vi "Up_PatternMatch.vi"(0 "Image In":T4, 2 "Template Image":T4, 5 "ROIIn":string, 11 "error in":errorcluster) -> (3 "Match":T1, 4 "Image Out":T4, 6 "Result":T3, 8 "ResultShow":T2, 10 "OK":bool, 14 "resulting string":string, 15 "error out":errorcluster)   [LabVIEW 2019]
uses:
  <vilib>/vision/Image Controls.llb/IMAQ Image.ctl
  <vilib>/vision/NI_Vision_Development_Module.lvlib
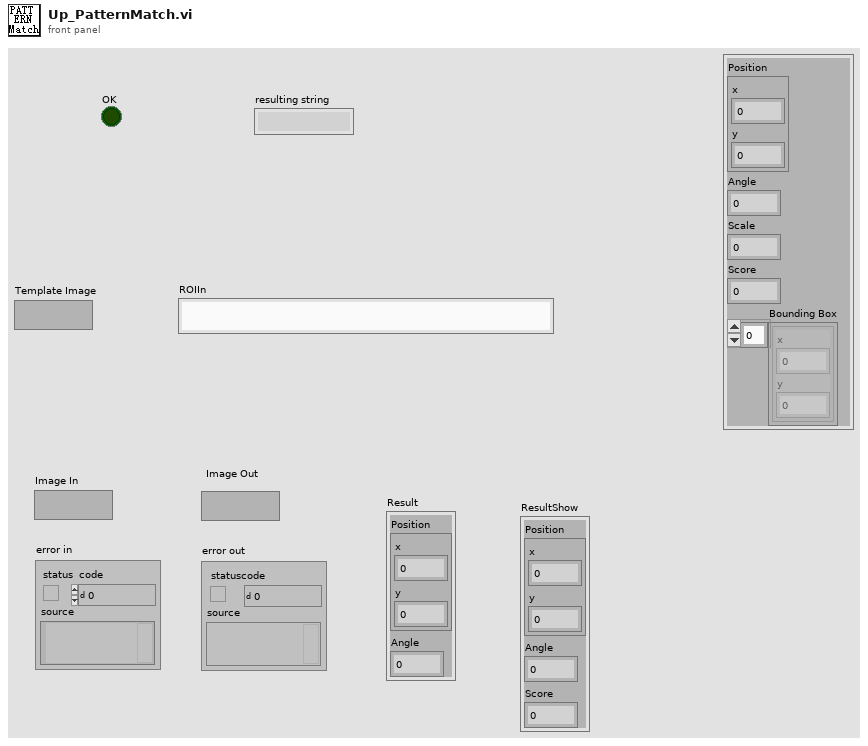
[diagram p1: front panel]
types:
  T1 = cluster{"Position":cluster{"x":sgl, "y":sgl}, "Angle":sgl, "Scale":sgl, "Score":sgl, "Bounding Box":cluster{"x":sgl, "y":sgl}[]}
  T2 = cluster{"Position":cluster{"x":sgl, "y":sgl}, "Angle":sgl, "Score":sgl}
  T3 = cluster{"Position":cluster{"x":sgl, "y":sgl}, "Angle":sgl}
  T4 = typedef "IMAQ Image.ctl" = refnum<image>
  T5 = typedef "IMAQ Rectangle" = cluster{"Left":i32, "Top":i32, "Right":i32, "Bottom":i32, "Rotation":dbl}
  T6 = cluster{"Number of Matches Requested":i32, "Minimum Match Score":sgl, "Angle Ranges":cluster{"Start Angle":sgl, "End Angle":sgl}[]}
  T7 = typedef "Image Type" = u32
  T8 = typedef "ROI Descriptor" = cluster{"Global Rectangle":i32[], "Contours":cluster{"ID":enum32{"External", "Internal"}, "Type":u32, "Coordinates":i32[]}[]}
  T9 = cluster{"Position":cluster{"x":sgl, "y":sgl}, "Angle":sgl, "Scale":sgl, "Score":sgl, "Bounding Box":cluster{"x":sgl, "y":sgl}[]}[]
  T10 = cluster{"Position":cluster{"x":sgl, "y":sgl}, "Angle":sgl, sgl}
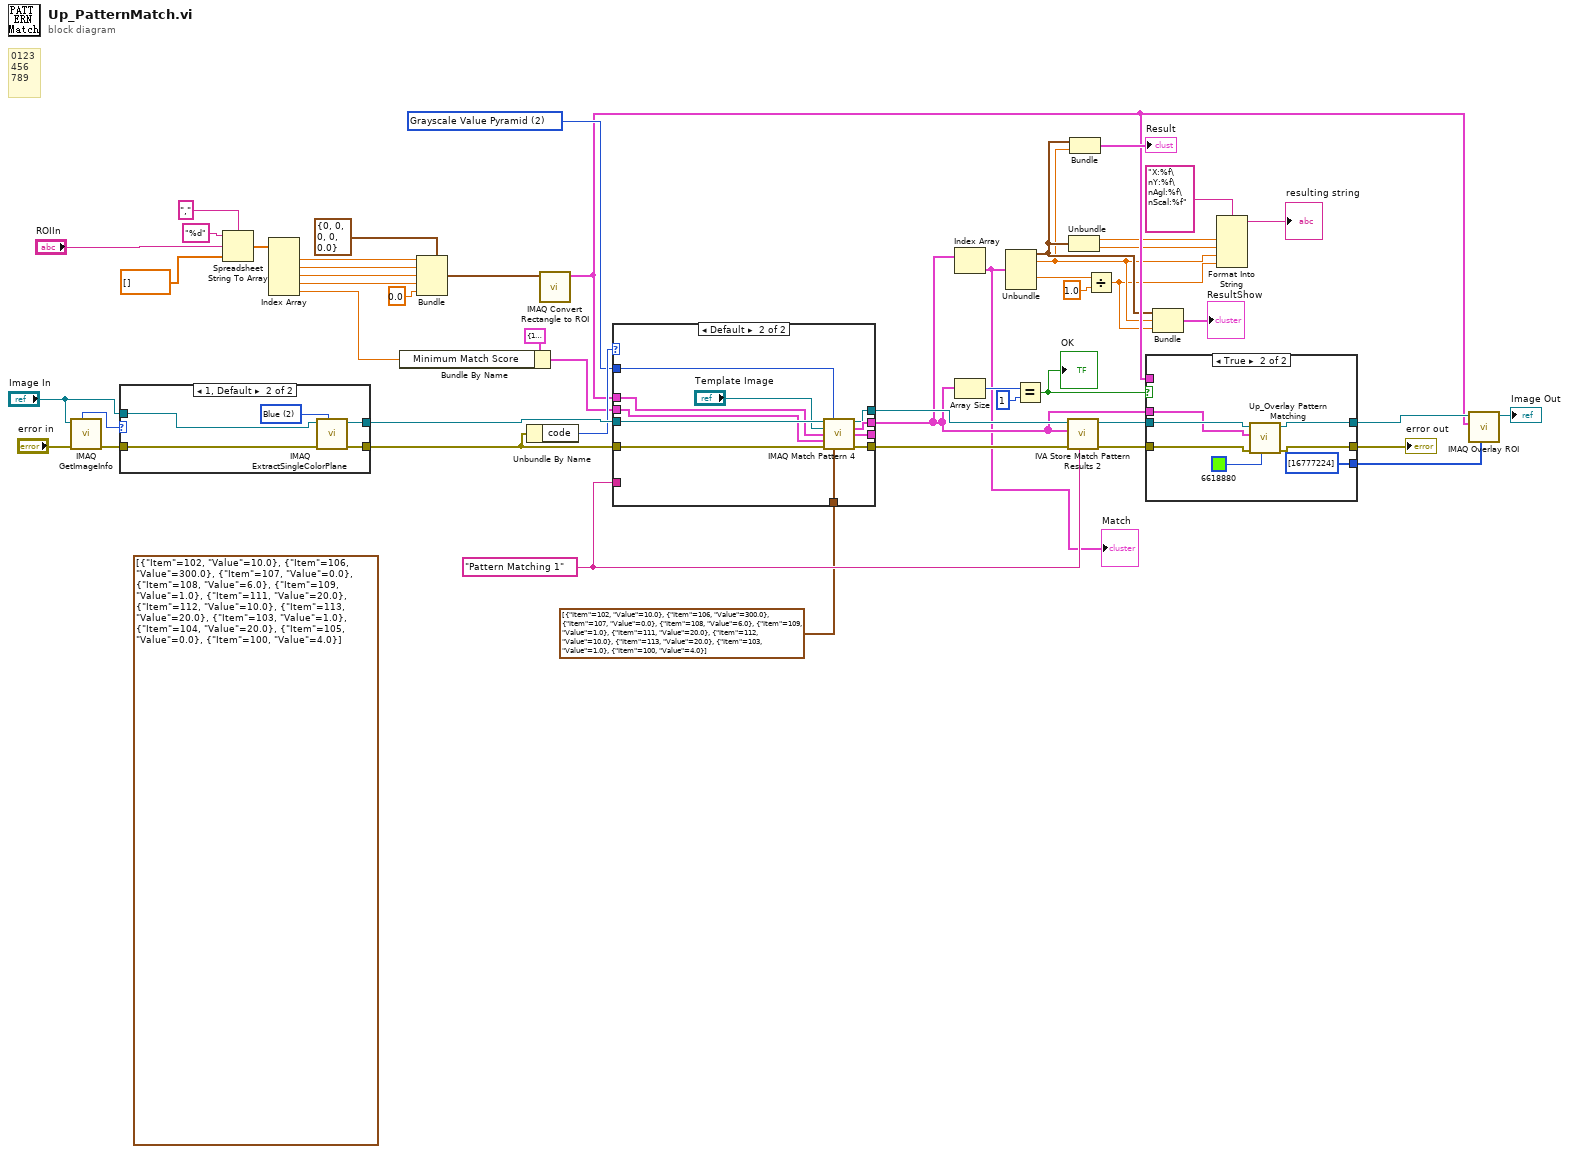
[diagram p0: block diagram]
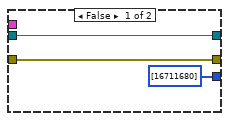
[diagram p3: hidden frame]
diagram:
  (unwired) cluster{"Item":u16, "Value":dbl}[] [{"Item"=102, "Value"=10.0}, {"Item"=106, "Value"=300.0}, {"Item"=107, "Value"=0.0}, {"Item"=108, "Value"=6.0}, {"Item"=109, "Value"=1.0}, {"Item"=111, "Value"=20.0}, {"Item"=112, "Value"=10.0}, {"Item"=113, "Value"=20.0}, {"Item"=103, "Value"=1.0}, {"Item"=104, "Value"=20.0}, {"Item"=105, "Value"=0.0}, {"Item"=100, "Value"=4.0}] ("Advanced Options")
  w27 = 2 items=["All", "Low Discrepancy Sampling", "Grayscale Value Pyramid", "Gradients Pyramid"] ("Algorithm")
  w45 = "Pattern Matching 1" ("Step Name")
  # "0123\n456\n789"
  n1 = call "IMAQ GetImageInfo"("error in (no error)"="error in", "Image"="Image In") -> ("error out"=w29:errorcluster, "Image Type"=w30:T7)  [unwired: 2 in, 6 out]
  n2 = case shown="1, Default" w30 {
    tunnel: [w51 w57] -> w50
    tunnel: [w52 w56] -> w49
    tunnel: w29 -> [w51 w55]
    tunnel: "Image In" -> [w52 w54]
    frame 0 {
    }
    frame 1, Default {
      w53 = 2 items=["Red", "Green", "Blue", "Hue", "Saturation", "Luminance", "Value", "Intensity"] ("Color Plane")
      n3 = call "IMAQ ExtractSingleColorPlane"("Color Plane"=w53, "error in (no error)"=w55, "Image Src"=w54) -> ("error out"=w57:errorcluster, "Image Dst Out"=w56:T4)  [unwired: 1 in, 6 out]
    }
  }
  n4 = Spreadsheet String To Array(delimiter (Tab)=",", format string="%d", spreadsheet string="ROIIn", array type (2D Dbl)=dbl[] []) -> (array=w10:dbl[])
  n5 = Index Array(array=w10) -> (element #1=w9:dbl, element #2=w8:dbl, element #3=w7:dbl, element #4=w6:dbl, element #5=w4:dbl)  [unwired: 5 in]
  n6 = Bundle By Name(cluster=T6 {"Number of Matches Requested"=1, "Minimum Match Score"=800.0, "Angle Ranges"=[]} ("Parameters"), "Minimum Match Score"=w4) -> (w39:T6)
  n7 = Bundle(cluster=T5 {"Left"=0, "Top"=0, "Right"=0, "Bottom"=0, "Rotation"=0.0} ("Rectangle"), "Left"=w9, "Top"=w8, "Right"=w7, "Bottom"=w6, "Rotation"=0.0) -> (w11:T5)
  n8 = Unbundle By Name(w50) -> ("code"=w46:i32)
  n9 = call "IMAQ Convert Rectangle to ROI"("Rectangle"=w11) -> ("ROI Descriptor"=w23:T8)  [unwired: 8 in, 1 out]
  n10 = case shown="Default" w46 {
    tunnel: w50 -> [_ w62]
    tunnel: w49 -> [w58 w67]
    tunnel: [_ w68] -> w48
    tunnel: [_ w69] -> w3
    tunnel: [w58 w66] -> w47
    tunnel: w45 -> [_ _]
    tunnel: w27 -> [_ w60]
    tunnel: w23 -> [_ w65]
    tunnel: w39 -> [_ w64]
    tunnel: [_ w63] -> _
    tunnel: cluster{"Item":u16, "Value":dbl}[] [{"Item"=102, "Value"=10.0}, {"Item"=106, "Value"=300.0}, {"Item"=107, "Value"=0.0}, {"Item"=108, "Value"=6.0}, {"Item"=109, "Value"=1.0}, {"Item"=111, "Value"=20.0}, {"Item"=112, "Value"=10.0}, {"Item"=113, "Value"=20.0}, {"Item"=103, "Value"=1.0}, {"Item"=100, "Value"=4.0}] ("Advanced Options") -> [_ w59]
    frame -1074396199, -1074396198 {
      # "Discard Coordinate System Error"
    }
    frame Default {
      n11 = call "IMAQ Match Pattern 4"("Image"=w67, "Algorithm"=w60, "Template Image"="Template Image", "ROI Descriptor"=w65, "Parameters"=w64, "error in (no error)"=w62, "Advanced Options"=w59) -> ("Image (duplicate)"=w66:T4, "Matches (pixel)"=w69:T9, "Matches (real-world)"=w63:T9, "error out"=w68:errorcluster)  [unwired: 4 in, 1 out]
    }
  }
  n12 = Index Array(array=w3) -> (element=w2:T1)  [unwired: 1 in]
  "Match" <- w2
  n13 = Array Size(array=w3) -> (size(s)=w35:i32)
  n14 = Unbundle(w2) -> ("Position"=w18:cluster{"x":sgl, "y":sgl}, "Angle"=w15:sgl, "Score"=w22:sgl)  [unwired: 2 out]
  n15 = Equal?(x=w35, y=1) -> (x = y?=w33:bool)
  "OK" <- w33
  n16 = call <vilib>:"IVA Store Match Pattern Results 2.vi"("Step Name"=w45, "error in (no error)"=w48, "Matches (pixel)"=w3, "Image in"=w47) -> ("error out"=w37:errorcluster, "Image dup"=w38:T4)  [unwired: 2 in, 4 out]
  n17 = Unbundle(w18) -> ("x"=w17:sgl, "y"=w16:sgl)
  n18 = Bundle("Position"=w18, "Angle"=w15) -> (→"Result":T3)  [unwired: 1 in]
  n19 = Divide(x=w22, y=sgl 1.0) -> (x/y=w14:sgl)
  n20 = case shown="True" w33 {
    tunnel: w38 -> [w72 w78]
    tunnel: [w72 w77] -> w25
    tunnel: w3 -> [_ w74]
    tunnel: w37 -> [w71 w75]
    tunnel: [w71 w73] -> w36
    tunnel: w23 -> [_ _]
    tunnel: [u32[] [16711680] ("Colors (Green)") u32[] [16777224] ("Colors (Green)")] -> w26
    frame False {
    }
    frame True {
      n21 = call "Up_Overlay Pattern Matching.vi"("Color"=u32 6618880, "error in"=w75, "Matches"=w74, "Image"=w78) -> ("error out"=w73:errorcluster, "Image Out"=w77:T4)  [unwired: 6 in]
    }
  }
  "error out" <- w36
  n22 = Bundle("Position"=w18, "Angle"=w15, w14) -> (→"ResultShow":T10)  [unwired: 1 in]
  n23 = Format Into String(format string="X:%f\nY:%f\nAgl:%f\nScal:%f", w17, w16, w15, w14) -> (resulting string=→"resulting string":string)  [unwired: 2 in, 1 out]
  n24 = call "IMAQ Overlay ROI"("Colors (Green)"=w26, "ROI Descriptor"=w23, "Image"=w25) -> ("Image Out"=→"Image Out":T4)  [unwired: 7 in, 1 out]
